vi "Initialize.vi"(4 "EXTERNAL MICROCONTROLLER":refnum<visa-resource-name>, 5 "String":string, 6 "dup Message Queue":refnum<queue>, 7 "Apply":bool, 8 "error in (no error)":errorcluster, 9 "GRBL COM PORT":refnum<visa-resource-name>, 10 "Tab Control":refnum<vi>, 11 "TabControl in":refnum<vi>) -> (0 "error out":errorcluster, 2 "Cluster":T1, 3 "APN REVISION NUMBER":string)   [LabVIEW 2021]
uses:
  support/Message Queue/Message Cluster.ctl
  support/Message Queue/Enqueue Message (Single).vi
  support/Message Queue/Message Queue.lvlib
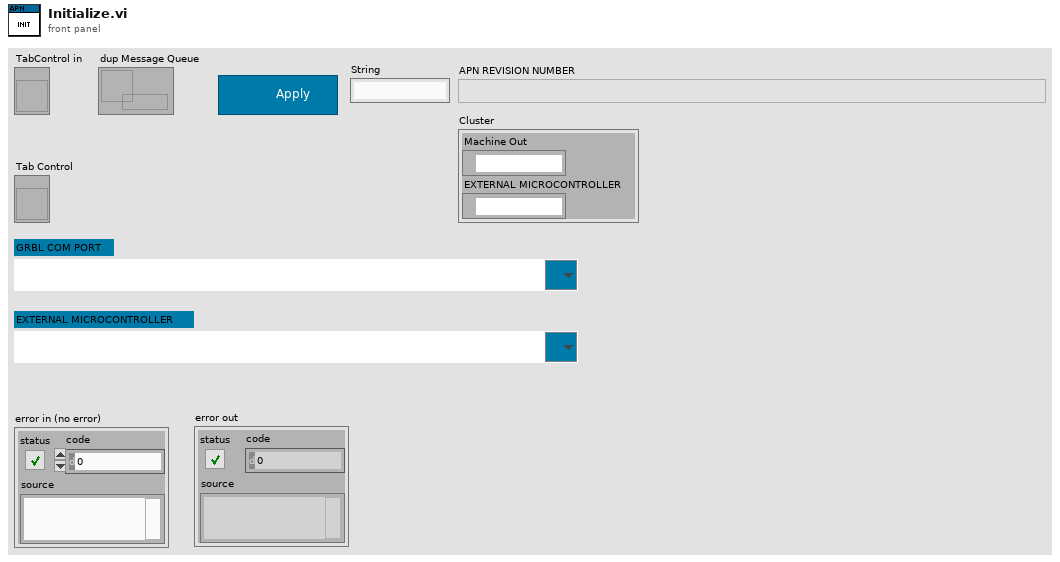
[diagram p1: front panel]
types:
  T1 = cluster{"Machine Out":refnum<visa-resource-name>, "EXTERNAL MICROCONTROLLER":refnum<visa-resource-name>}
  T2 = enum32{"Serial Configuration", "GCODE", "Manual Overide", "Tune"}
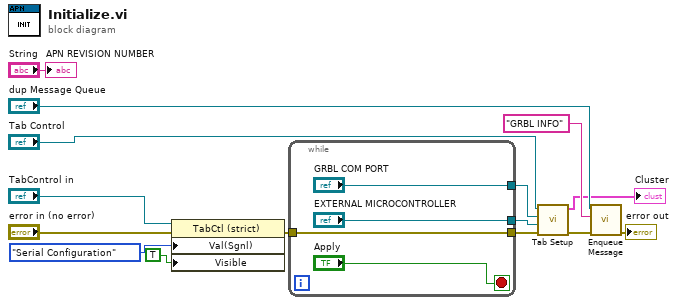
[diagram p0: block diagram]
diagram:
  n1 = property on="Property Node" class="TabCtl (strict)"(reference="TabControl in", error in="error in (no error)", "Val(Sgnl)"=T2."Serial Configuration" ("Value (Signaling)"), "Visible"=TRUE) -> (error out=w5:errorcluster)  [unwired: 1 out]
  n2 = while {
    tunnel: w5 -> [w18]
    tunnel: [w18] -> w6
    tunnel: ["GRBL COM PORT"] -> w7
    tunnel: ["EXTERNAL MICROCONTROLLER"] -> w8
    stop <- "Apply" stop-if-true
  }
  n3 = call "Tab Setup.vi"("error in (no error)"=w6, "EXTERNAL MICROCONTROLLER"=w8, "GRBL COM PORT"=w7, "TabControl in"="Tab Control") -> ("error out"=w13:errorcluster, "Cluster"=→"Cluster":T1)  [unwired: 6 in]
  n4 = call-poly "Enqueue Message.vi"("error in (no error)"=w13, "Message"="GRBL INFO", "Message Queue"="dup Message Queue") -> ("error out"=→"error out":errorcluster)  [unwired: 7 in, 1 out]
  "APN REVISION NUMBER" <- "String"
